vi "SW_Gen_Get_Initial_picture_Scaling_and_Cage_size.vi"(8 "Diameter of the cage, mm":dbl=180.0 format="%#_13g", 9 "Scale factor for outer display radius display":dbl=0.95 format="%#_13g", 10 "Background color":u32(colorbox)=13816530, 11 "Draw Area Size":cluster{"Width":dbl, "Height":dbl}={"Width"=480.0, "Height"=480.0}) -> (0 "Pixels per mm":dbl, 1 "Fonts scale factor":dbl, 2 "Radius of displayed outer segments, pix":dbl, 3 "Zones display background":picture)   [LabVIEW 2016]
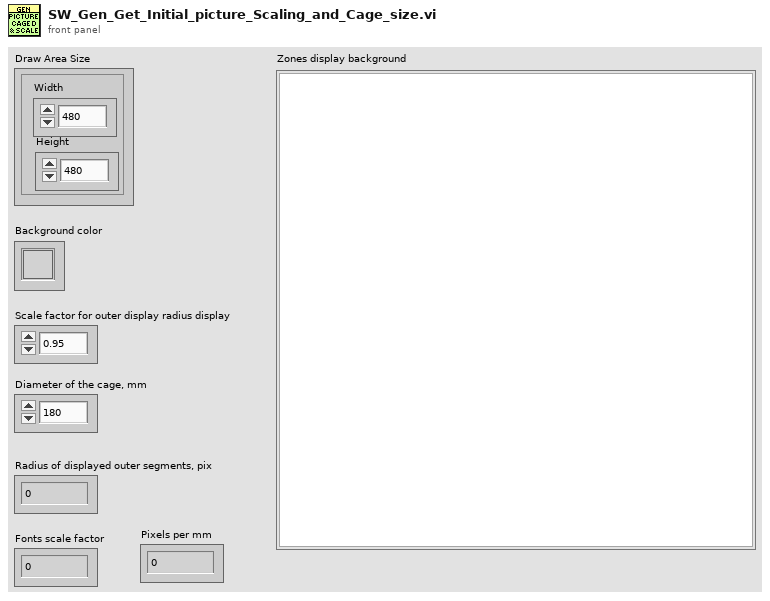
[diagram p1: front panel]
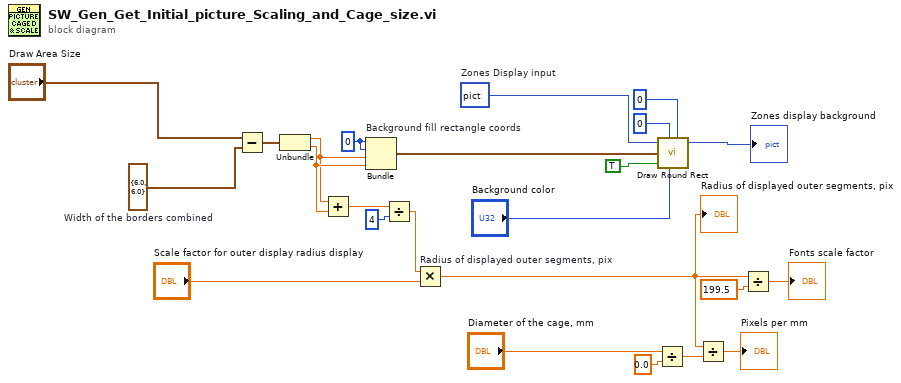
[diagram p0: block diagram]
diagram:
  w9 = cluster{"Width":dbl, "Height":dbl} {"Width"=6.0, "Height"=6.0}  # Width of the borders combined
  w21 = picture data[5B]  # Zones Display input
  w6 = 0
  n1 = Subtract(x="Draw Area Size", y=w9) -> (x-y=w7:cluster{"Width":dbl, "Height":dbl})
  n2 = Unbundle(w7) -> ("Width"=w16:dbl, "Height"=w17:dbl)
  n3 = Add(x=w16, y=w17) -> (x+y=w15:dbl)
  n4 = Bundle "Background fill rectangle coords"(w6, w6, "Width"=w16, "Height"=w17) -> (w22:cluster{i32, i32, "Width":dbl, "Height":dbl})  [unwired: 1 in]
  n5 = Divide(x=w15, y=u32 4) -> (x/y=w12:dbl)
  n6 = Multiply "Radius of displayed outer segments, pix"(x=w12, y="Scale factor for outer display radius display") -> (x*y=w3:dbl)
  "Radius of displayed outer segments, pix" <- w3
  n7 = Divide(x="Diameter of the cage, mm", y=0.0) -> (x/y=w2:dbl)
  n8 = call <vilib>:"Draw Round Rect.vi"("picture"=w21, "oval width"=i16 0, "rect"=w22, "fill?(F)"=TRUE, "color(black)"="Background color", "oval height"=i16 0) -> ("new picture"=→"Zones display background":picture)  [unwired: 3 in]
  n9 = Divide(x=w3, y=w2) -> (x/y=→"Pixels per mm":dbl)
  n10 = Divide(x=w3, y=199.5) -> (x/y=→"Fonts scale factor":dbl)
